vi "create slopes paths.vi"(10 "Strip Path":bool, 11 "Path":path=path "C:/Cascade/Data/Output Files/slopes-cal-record.csv") -> (2 "Record Output Slopes for slopes.csv File":path, 3 "Record Output Slopes to  Record File":path)   [LabVIEW 2016]
uses:
  <userlib>/_OpenG.lib/file/file.llb/Strip Path - Traditional__ogtk.vi
  <userlib>/_OpenG.lib/file/file.llb/Build Path - Traditional__ogtk.vi
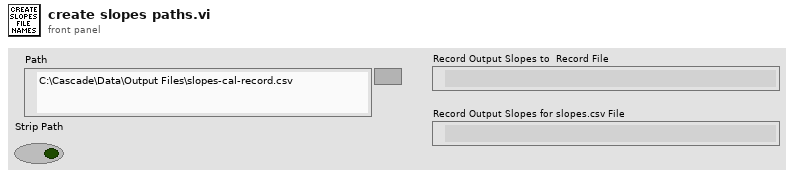
[diagram p1: front panel]
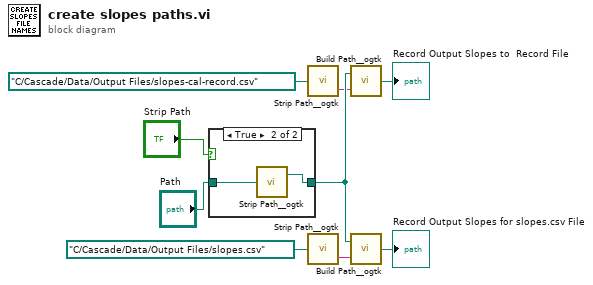
[diagram p0: block diagram]
diagram:
  n1 = case shown="True" "Strip Path" {
    tunnel: "Path" -> [w10 w12]
    tunnel: [w10 w11] -> w5
    frame False {
    }
    frame True {
      n2 = call-poly <userlib>:"Strip Path__ogtk.vi"("path"=w12) -> ("stripped path"=w11:path)  [unwired: 1 out]
    }
  }
  n3 = call-poly <userlib>:"Strip Path__ogtk.vi"("path"=path "C:/Cascade/Data/Output Files/slopes-cal-record.csv") -> ("name"=w3:string)  [unwired: 1 out]
  n4 = call-poly <userlib>:"Strip Path__ogtk.vi"("path"=path "C:/Cascade/Data/Output Files/slopes.csv") -> ("name"=w6:string)  [unwired: 1 out]
  n5 = call-poly <userlib>:"Build Path__ogtk.vi"("name or relative path"=w3, "base path"=w5) -> ("appended path"=→"Record Output Slopes to  Record File":path)
  n6 = call-poly <userlib>:"Build Path__ogtk.vi"("name or relative path"=w6, "base path"=w5) -> ("appended path"=→"Record Output Slopes for slopes.csv File":path)
